vi "MDAQ_Parse_Sum.vi"(8 "error in":errorcluster, 10 "input buffer":string) -> (0 "error out":errorcluster, 2 "Sum":u32)   [LabVIEW 2021]
uses:
  <vilib>/regexp/Match Regular Expression.xnode
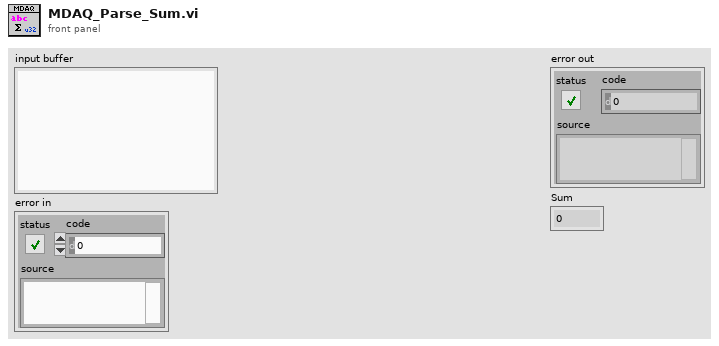
[diagram p1: front panel]
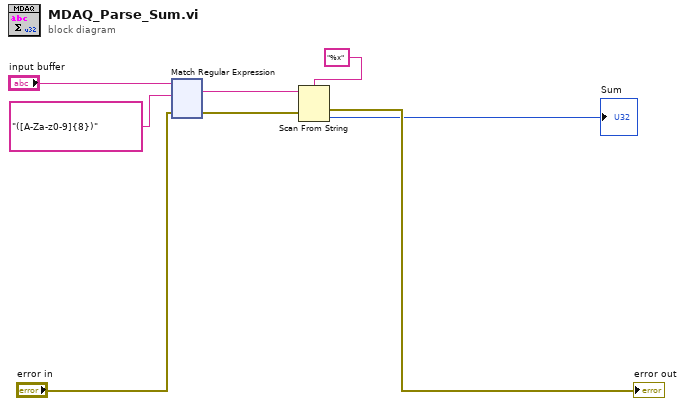
[diagram p0: block diagram]
diagram:
  n1 = xnode "Match Regular Expression"("input string"="input buffer", "regular expression"="([A-Za-z0-9]{8})", "error in"="error in") -> ("whole match"=w5:string, "error out"=w4:errorcluster)  [unwired: 3 in, 3 out]
  n2 = Scan From String(format string="%x", input string=w5, error in=w4) -> (error out=→"error out":errorcluster, output 1=→"Sum":u32)  [unwired: 2 in, 2 out]
